vi "Get DIO Logic Thresholds.vi"(8 "error in (no error)":errorcluster, 11 "DIO Board Ref in":T1 format="%.0x") -> (0 "error out":errorcluster, 1 "Ordered DIO Channels":T1[](array[typedef]) format="%.0x", 2 "Logic Thresholds":dbl[](array[numeric]), 3 "DIO Board Ref out":T1 format="%.0x")   [LabVIEW 2014, in "SLSC configuration System Explorer.lvlib"]
doc: "Orders the fault channels and gets the current fault states of a single FIU board."
uses:
  SLSC configuration System Explorer.lvlib
  <vilib>/NI Veristand/Custom Device API/Custom Device Item Ref.ctl
  Shared/Constants.vi
  <vilib>/NI Veristand/Custom Device API/Get Item Property (U16).vi
  <vilib>/NI Veristand/Custom Device API/Custom Device API.lvlib
  Shared/SLSC configuration Shared.lvlib
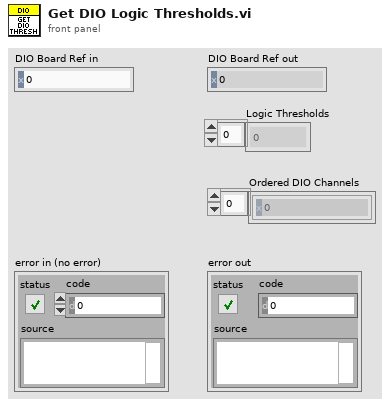
[diagram p1: front panel]
types:
  T1 = typedef "Custom Device API.lvlib/Custom Device Item Ref.ctl" = u64
  T2 = typedef "Custom Device API.lvlib/Custom Device Channel.ctl" = cluster{"Type":T3, "Units":string, "Default Value":dbl, "Faultable":bool, "Scalable":bool}
  T3 = typedef "Custom Device API.lvlib/Custom Device Channel Type.ctl" = enum16{"Input", "Output"}
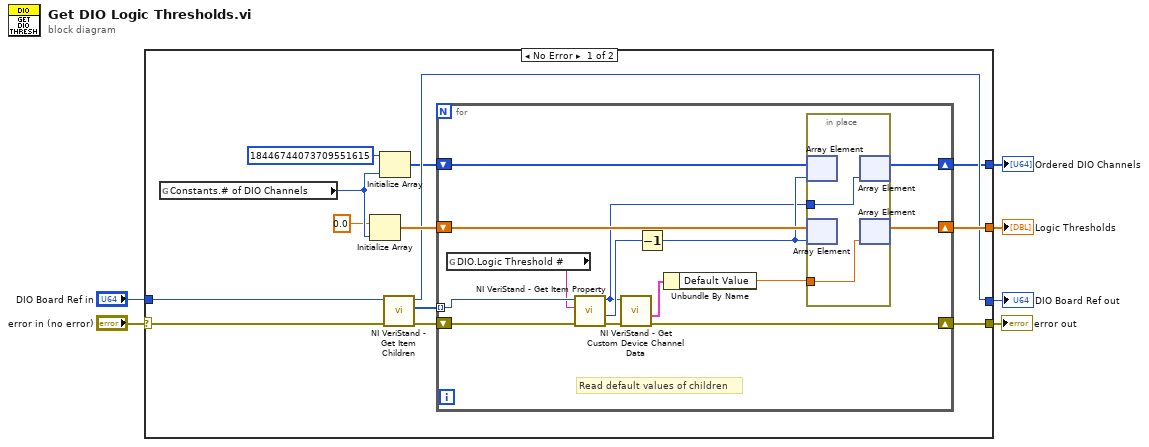
[diagram p0: block diagram]
diagram:
  n1 = case shown="No Error" "error in (no error)" {
    selector: "error in (no error)" -> [w13 w36]
    tunnel: "DIO Board Ref in" -> [w18 w37]
    tunnel: [w17 w36] -> w5
    tunnel: [w14 _] -> w1
    tunnel: [w12 w37] -> w3
    tunnel: [w8 _] -> w2
    frame No Error {
      n2 = global read "Constants.vi" "Constants.# of DIO Channels"() -> (w10:u8)
      n3 = Initialize Array(0.0, w10) -> (w19:dbl[])
      n4 = Initialize Array(T1 18446744073709551615 ("Item Ref out"), w10) -> (w9:T1[])
      n5 = call <vilib>:"NI VeriStand - Get Item Children.vi"("error in (no error)"=w13, "Item Ref in"=w18) -> ("error out"=w16:errorcluster, "Child Refs"=w15:T1[], "Item Ref out"=w12:T1)  [unwired: 6 in, 1 out]
      n6 = for {
        tunnel: w15 -> [w33] mode=indexing
        shift-right: [w26] -> w17
        shift-left: w16 -> [w31]
        shift-right: [w25] -> w14
        shift-left: w19 -> [w27]
        shift-right: [w21] -> w8
        shift-left: w9 -> [w24]
        # "Read default values of children"
        n7 = global read "Constants.vi" "DIO.Logic Threshold #"() -> (w32:string)
        n8 = call-poly <vilib>:"NI VeriStand - Get Item Property.vi"("error in (no error)"=w31, "Property Name"=w32, "Item Ref in"=w33) -> ("error out"=w29:errorcluster, "Value"=w30:u16, "Item Ref out"=w22:T1)  [unwired: 5 in, 1 out]
        n9 = call <vilib>:"NI VeriStand - Get Custom Device Channel Data.vi"("error in (no error)"=w29, "Channel Ref in"=w22) -> ("error out"=w26:errorcluster, "Channel"=w28:T2)  [unwired: 4 in, 4 out]
        n10 = Decrement(x=w30) -> (x-1=w23:u16)
        n11 = Unbundle By Name(w28) -> ("Default Value"=w20:dbl)
        n12 = in-place {
          in-place-border: w20 -> [w35]
          in-place-border: w22 -> [w34]
          n13 = in-place-array #1(w24, w23) -> ()  [unwired: 1 out]
          n14 = in-place-array #2(w27, w23) -> ()  [unwired: 1 out]
          n15 = in-place-array #1(w34) -> (w21:T1[])  [unwired: 1 out]
          n16 = in-place-array #2(w35) -> (w25:dbl[])  [unwired: 1 out]
        }
      }
    }
    frame Error {
    }
  }
  "error out" <- w5
  "DIO Board Ref out" <- w3
  "Ordered DIO Channels" <- w2
  "Logic Thresholds" <- w1
